vi "testItem.vi"(8 "error in (no error)":errorcluster, 11 "TestCase in":refnum<class "ObjectList_Delegations.lvclass">) -> (0 "error out":errorcluster, 3 "TestCase out":refnum<class "ObjectList_Delegations.lvclass">)   [LabVIEW 2013, in "ObjectList_Delegations.lvclass"]
uses:
  ObjectList_Delegations.lvclass
  ObjectList_Delegations.lvclass/ObjectList_Delegations.ctl
  source/LapDog.Collections.Lists/ObjectList/ObjectList.lvclass
  <vilib>/addons/_JKI Toolkits/VI Tester/TestCase.llb/TestCase.lvclass
  UnitTestComparisons/UnitTestComparisons.lvlib
  Test Doubles/ListImp_RefSpy/ListImp_RefSpy.lvclass
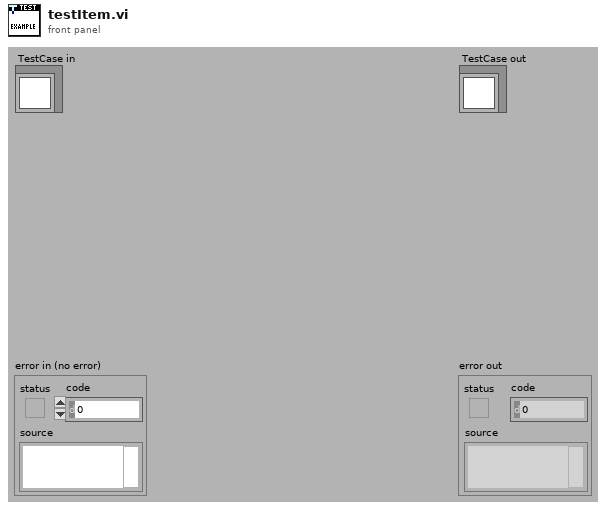
[diagram p1: front panel]
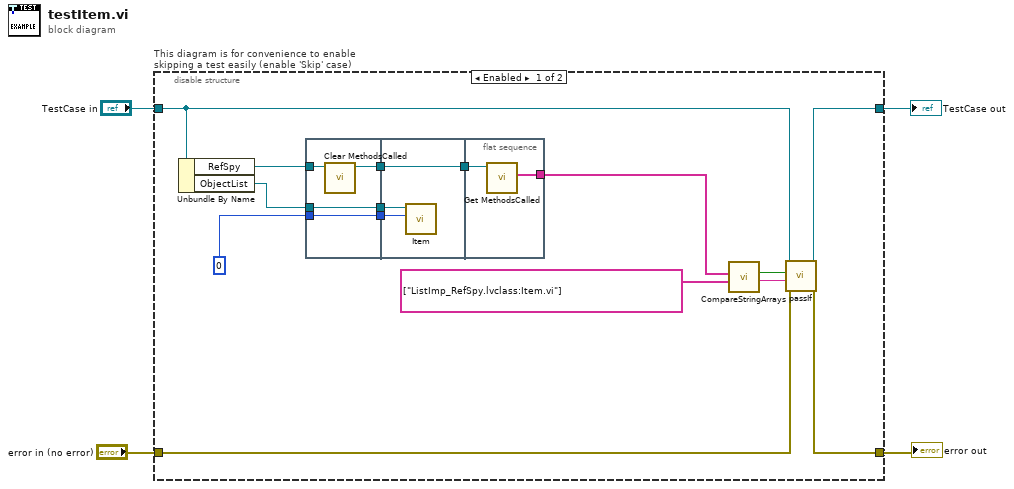
[diagram p0: block diagram]
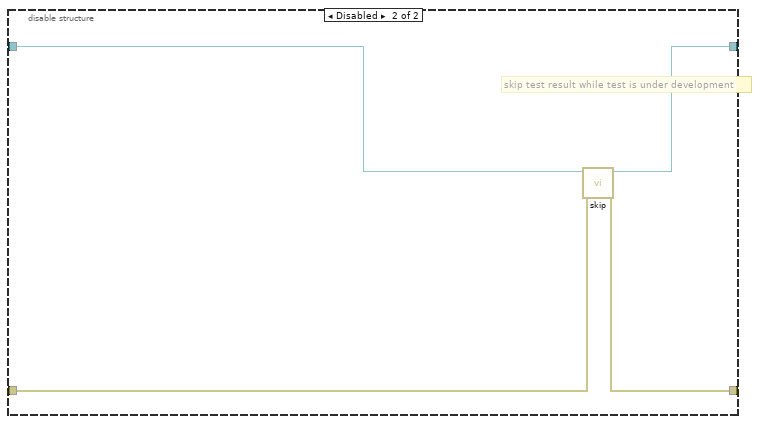
[diagram p2: hidden frame]
diagram:
  n1 = disable-structure "This diagram is for convenience to enable skipping a test easily (enable 'Skip' case)" shown="Enabled" {
    disable-tunnel: "TestCase in" -> [w14 w32]
    disable-tunnel: [w19 w30] -> w1
    disable-tunnel: [w18 w31] -> w3
    disable-tunnel: "error in (no error)" -> [w17 w29]
    frame Enabled {
      n2 = Unbundle By Name(w14) -> ("RefSpy"=w11:refnum<class "ListImp_RefSpy.lvclass">, "ObjectList"=w13:refnum<class "ObjectList.lvclass">)
      n3 = flat-sequence {
        tunnel: w11 -> [w22]
        tunnel: w13 -> [w23]
        tunnel: [w23] -> w8
        tunnel: [w21] -> w7
        tunnel: 0 -> [w20]
        tunnel: [w20] -> w5
        tunnel: [w26] -> w12
        tunnel: w8 -> [w25]
        tunnel: w7 -> [w26]
        tunnel: w5 -> [w24]
        tunnel: w12 -> [w28]
        tunnel: [w27] -> w9
        frame #0 {
          n4 = call "Clear MethodsCalled.vi"("MockListImp in"=w22) -> ("MockListImp out"=w21:refnum<class "ListImp_RefSpy.lvclass">)  [unwired: 9 in, 1 out]
        }
        frame #1 {
          n5 = call-dynamic "Item.vi"("Index"=w24, "List in"=w25) -> ()  [unwired: 7 in, 3 out]
        }
        frame #2 {
          n6 = call "Get MethodsCalled.vi"("MockListImp"=w28) -> ("MethodsCalled"=w27:string[])  [unwired: 9 in, 1 out]
        }
      }
      n7 = call "CompareStringArrays.vi"("Expected Strings"=string[] ["ListImp_RefSpy.lvclass:Item.vi"] ("Actual Strings"), "Actual Strings"=w9) -> ("Message"=w15:string, "Equal?"=w16:bool)  [unwired: 8 in]
      n8 = call-dynamic "passIf.vi"("error in (no error)"=w17, "message (\"\")"=w15, "pass"=w16, "TestCase in"=w14) -> ("error out"=w18:errorcluster, "TestCase out"=w19:refnum<class "ObjectList_Delegations.lvclass">)  [unwired: 6 in]
    }
    frame Disabled {
      # "skip test result while test is under development"
      n9 = call <vilib>:"skip.vi"("error in (no error)"=w29, "TestCase in"=w32) -> ("error out"=w31:errorcluster, "TestCase out"=w30:refnum<class "ObjectList_Delegations.lvclass">)  [unwired: 8 in]
    }
  }
  "error out" <- w3
  "TestCase out" <- w1
